vi "Init.vi"(8 "error in":errorcluster, 11 "Fgen PXI CFG in":refnum<class "Fgen PXI CFG.lvclass">) -> (0 "error out":errorcluster, 3 "Fgen PXI CFG out":refnum<class "Fgen PXI CFG.lvclass">)   [LabVIEW 2023, in "HAL.lvlib" / "Fgen PXI.lvlib" / "Fgen PXI CFG.lvclass"]
uses:
  Fgen PXI CFG.lvclass
  Fgen PXI CFG.lvclass/Fgen PXI CFG.ctl
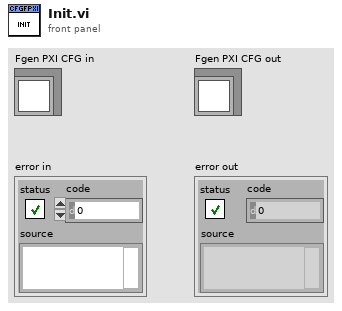
[diagram p1: front panel]
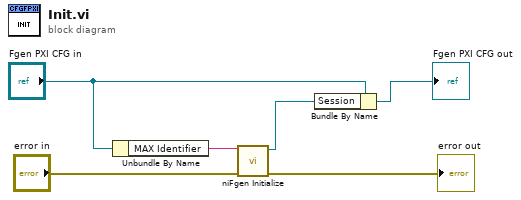
[diagram p0: block diagram]
diagram:
  n1 = Unbundle By Name("Fgen PXI CFG in") -> ("MAX Identifier"=w6:string)
  n2 = call <instrlib>:"niFgen Initialize.vi"("error in (no error)"="error in", "Resource Name"=w6) -> ("error out"=→"error out":errorcluster, "Instrument Handle Out"=w3:refnum<k15>)  [unwired: 8 in]
  n3 = Bundle By Name(cluster="Fgen PXI CFG in", "Session"=w3) -> (→"Fgen PXI CFG out":refnum<class "Fgen PXI CFG.lvclass">)
